vi "XYZStage-Increase or reduce speed setting.vi"(11 "Function":enum16{"Increase speed", "Reduce speed"}(ring)) -> ()   [LabVIEW 2020]
uses:
  Typedefs/XYZ stage states.ctl
  User Interface/Windows/Position control window/Globals/Pos ctrl window globals.vi
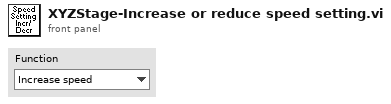
[diagram p1: front panel]
types:
  T1 = typedef "XYZ stage states.ctl" = enum16{"Dequeue", "Initialize", "Read Position", "Read Speed Setting", "Move", "Set Max Speed", "Reset Axis", "Stop all movement"}
  T2 = typedef "Pos Ctrl window refs cluster.ctl" = cluster{"menu reference":refnum<k9>, "X Coordinate ctrl":refnum<vi>, "Y Coordinate ctrl":refnum<vi>, "Z Coordinate ctrl":refnum<vi>, "Speed setting ctrl":refnum<vi>, "Up":refnum<vi>, "Down":refnum<vi>, "Left":refnum<vi>, "Right":refnum<vi>, "Z move up":refnum<vi>, "Z move down":refnum<vi>, "Down-left":refnum<vi>, "Down-right":refnum<vi>, "Up-left":refnum<vi>, "Up-right":refnum<vi>, "Step = size of image":refnum<vi>, "XY step (um)":refnum<vi>, "Z step (um)":refnum<vi>, "Speed setting\navailable":refnum<vi>}
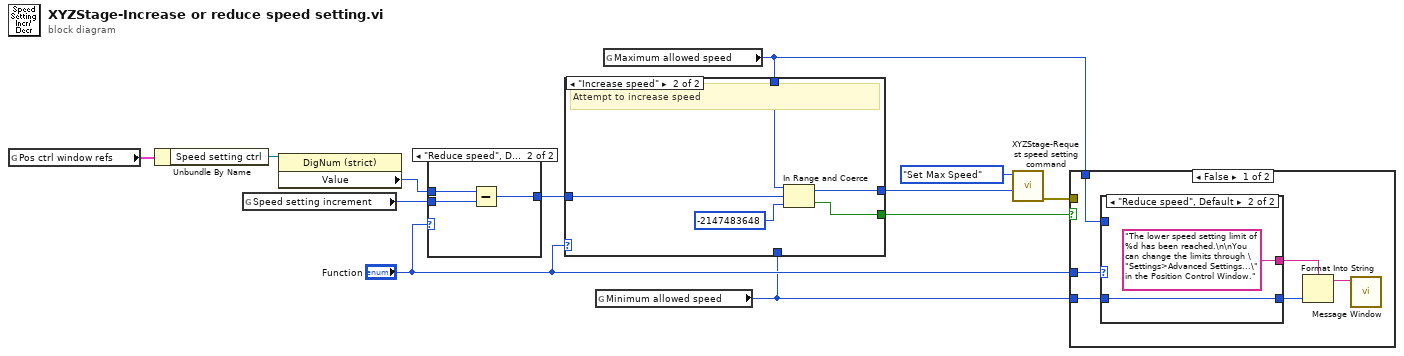
[diagram p0: block diagram]
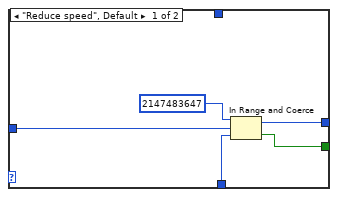
[diagram p2: hidden frame]
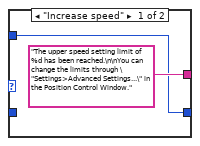
[diagram p3: hidden frame]
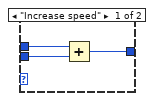
[diagram p5: hidden frame]
diagram:
  n1 = global read "Pos ctrl window globals.vi" "Pos ctrl window refs"() -> (w11:T2)
  n2 = Unbundle By Name(w11) -> ("Speed setting ctrl"=w12:refnum<vi>)
  n3 = global read "Pos ctrl window globals.vi" "Speed setting increment"() -> (w8:i32)
  n4 = property on="Property Node" class="DigNum (strict)"(reference=w12) -> ("Value"=w4:i32)  [unwired: 1 in, 2 out]
  n5 = case shown="\"Reduce speed\", Default" "Function" {
    tunnel: w8 -> [w15 w17]
    tunnel: [w14 w16] -> w5
    tunnel: w4 -> [w13 w18]
    frame "Increase speed" {
      n6 = Add(x=w13, y=w15) -> (x+y=w14:i32)
    }
    frame "Reduce speed", Default {
      n7 = Subtract(x=w18, y=w17) -> (x-y=w16:i32)
    }
  }
  n8 = global read "Pos ctrl window globals.vi" "Minimum allowed speed"() -> (w1:i32)
  n9 = global read "Pos ctrl window globals.vi" "Maximum allowed speed"() -> (w2:i32)
  n10 = case shown="\"Increase speed\"" "Function" {
    tunnel: [w23 w28] -> w10
    tunnel: [w21 w27] -> w7
    tunnel: w5 -> [w22 w26]
    tunnel: w1 -> [w19 _]
    tunnel: w2 -> [_ w24]
    frame "Reduce speed", Default {
      n11 = In Range and Coerce(upper limit=2147483647, x=w22, lower limit=w19) -> (coerced(x)=w23:i32, In Range?=w21:bool)
    }
    frame "Increase speed" {
      # "Attempt to increase speed"
      n12 = In Range and Coerce(upper limit=w24, x=w26, lower limit=-2147483648) -> (coerced(x)=w28:i32, In Range?=w27:bool)
    }
  }
  n13 = call "XYZStage-Request speed setting command.vi"("Speed to set"=w10, "Which speed setting command?"=XYZ_stage_states."Set Max Speed" ("Command")) -> ("Error Out (no error)"=w6:errorcluster)  [unwired: 9 in]
  n14 = case shown="False" w7 {
    tunnel: w6 -> [_ _]
    tunnel: "Function" -> [w34 _]
    tunnel: w2 -> [w31 _]
    tunnel: w1 -> [w29 _]
    frame False {
      n15 = case shown="\"Reduce speed\", Default" w34 {
        tunnel: ["The upper speed setting limit of %d has been reached.\n\nYou can change the limits through \"Settings>Advanced Settings...\" in the Position Control Window." ("Message string") "The lower speed setting limit of %d has been reached.\n\nYou can change the limits through \"Settings>Advanced Settings...\" in the Position Control Window." ("Message string")] -> w32
        tunnel: w31 -> [w35 _]
        tunnel: [w35 w37] -> w30
        tunnel: w29 -> [_ w37]
        frame "Increase speed" {
        }
        frame "Reduce speed", Default {
        }
      }
      n16 = Format Into String(format string=w32, w30) -> (resulting string=w33:string)  [unwired: 2 in, 1 out]
      n17 = call "Message Window.vi"("Message string"=w33) -> ()  [unwired: 10 in, 1 out]
    }
    frame True {
    }
  }
